vi "Sequence.GenerateSequence.vi"(8 "error in (no error)":errorcluster, 10 "output cluster":T1, 11 "Path":path) -> (0 "error out":errorcluster)   [LabVIEW 2013, in "Simple Sequence Editor.lvlib"]
uses:
  Simple Sequence Editor.lvlib
  Types/Compiled.RTSequenceProperties.ctl
  Types/ChannelProperties.ctl
  Types/Compiled.StepProperties.ctl
  Types/Compiled.StepElementProperties.ctl
  Types/StepTypes.ctl
  NationalInstruments.VeriStand.RealTimeSequenceDefinitionApi
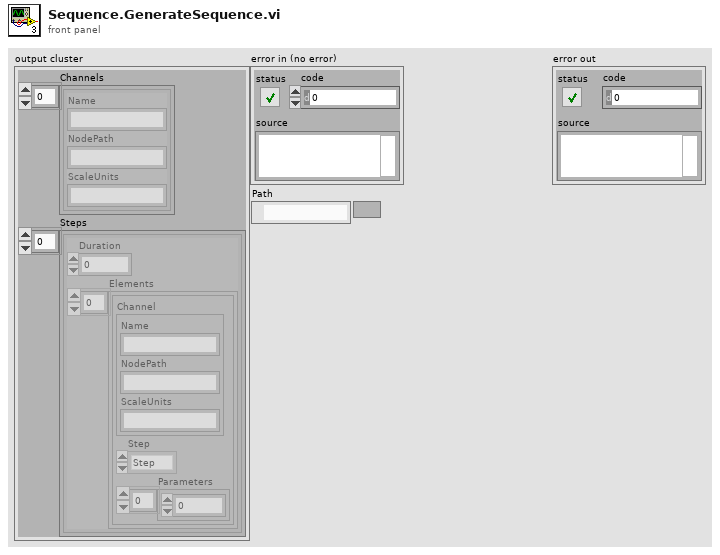
[diagram p1: front panel]
types:
  T1 = typedef "Simple Sequence Editor.lvlib/Compiled.RTSequenceProperties.ctl" = cluster{"Channels":T2[], "Steps":T3[]}
  T2 = typedef "Simple Sequence Editor.lvlib/ChannelProperties.ctl" = cluster{"Name":string, "NodePath":string, "ScaleUnits":string}
  T3 = typedef "Simple Sequence Editor.lvlib/Compiled.StepProperties.ctl" = cluster{"Duration":dbl, "Elements":T4[]}
  T4 = typedef "Simple Sequence Editor.lvlib/Compiled.StepElementProperties.ctl" = cluster{"Channel":T2, "Step":T5, "Parameters":dbl[]}
  T5 = typedef "Simple Sequence Editor.lvlib/StepTypes.ctl" = enum8{"Step", "iStep", "Ramp", "Unchanged", "Unknown"}
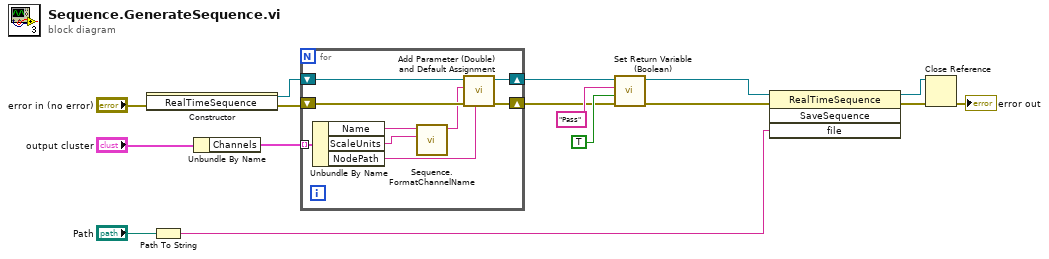
[diagram p0: block diagram]
diagram:
  n1 = constructor class="RealTimeSequence"(error in="error in (no error)") -> (reference out=w11:refnum<k24>, error out=w10:errorcluster)  [unwired: 2 in, 1 out]
  n2 = Path To String(path="Path") -> (string=w1:string)
  n3 = Unbundle By Name("output cluster") -> ("Channels"=w12:T2[])
  n4 = for {
    tunnel: w12 -> [w25] mode=indexing
    shift-right: [w18] -> w9
    shift-left: w10 -> [w21]
    shift-right: [w17] -> w8
    shift-left: w11 -> [w22]
    n5 = Unbundle By Name(w25) -> ("Name"=w24:string, "ScaleUnits"=w23:string, "NodePath"=w19:string)
    n6 = call "Sequence.FormatChannelName.vi"("ScaleUnits"=w23, "Name"=w24) -> ("String"=w20:string)  [unwired: 9 in]
    n7 = call "Add Parameter (Double) and Default Assignment.vi"("Default Assignment"=w19, "error in (no error)"=w21, "Identifier"=w20, "Sequence Ref in"=w22) -> ("error out"=w18:errorcluster, "Sequence Ref out"=w17:refnum<k24>)  [unwired: 6 in]
  }
  n8 = call "Set Return Variable (Boolean).vi"("error in (no error)"=w9, "Value"=TRUE, "Identifier"="Pass", "Sequence Ref in"=w8) -> ("error out"=w7:errorcluster, "Sequence Ref out"=w5:refnum<k24>)  [unwired: 6 in]
  n9 = invoke class="RealTimeSequence" method="SaveSequence"(reference=w5, error in=w7, "file"=w1) -> (reference out=w16:refnum<k24>, error out=w6:errorcluster)  [unwired: 1 in, 2 out]
  n10 = Close Reference(reference=w16, error in (no error)=w6) -> (error out=→"error out":errorcluster)
